vi "Process Data.vi"(8 "error in (no error)":errorcluster, 10 "AbstractData in":refnum<class "AbstractData.lvclass">, 11 "AbstractProcessor in":refnum<class "AbstractProcessor.lvclass">) -> (0 "error out":errorcluster, 2 "AbstractData out":refnum<class "AbstractData.lvclass">, 3 "AbstractProcessor out":refnum<class "AbstractProcessor.lvclass">)   [LabVIEW 2014, in "AbstractProcessor.lvclass"]
uses:
  AbstractProcessor.lvclass
  Model/Data/AbstractData/AbstractData.lvclass
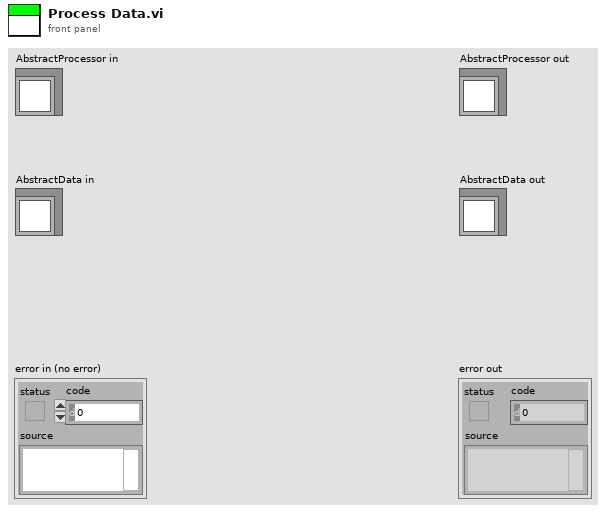
[diagram p1: front panel]
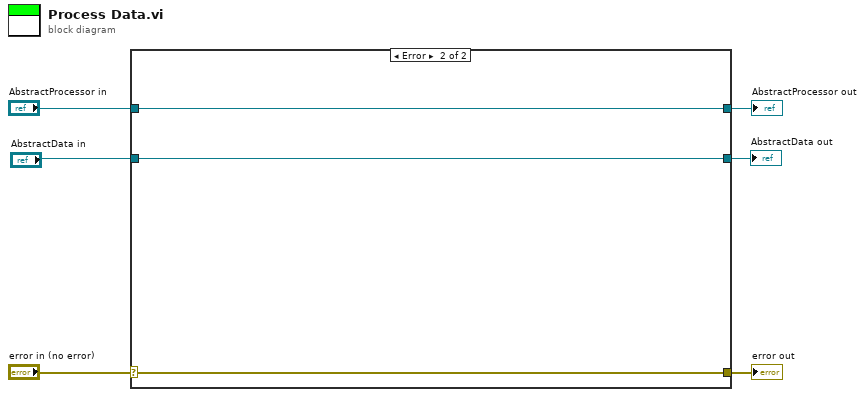
[diagram p0: block diagram]
diagram:
  n1 = case shown="Error" "error in (no error)" {
    selector: "error in (no error)" -> [w8 w12]
    tunnel: [w8 w12] -> w5
    tunnel: [w9 w11] -> w3
    tunnel: "AbstractProcessor in" -> [w9 w11]
    tunnel: "AbstractData in" -> [w7 w10]
    tunnel: [w7 w10] -> w1
    frame No Error {
      # "Wire the error cluster across even in the \"No Error\"\ncase so that warnings get propagated."
    }
    frame Error {
    }
  }
  "error out" <- w5
  "AbstractProcessor out" <- w3
  "AbstractData out" <- w1
